vi "SeCrTs-Obtain Message Queue_R.vi"(8 "error in (no error)":errorcluster) -> (0 "error out":errorcluster, 1 "Err Queue":refnum<queue>)   [LabVIEW 2022 SP3]
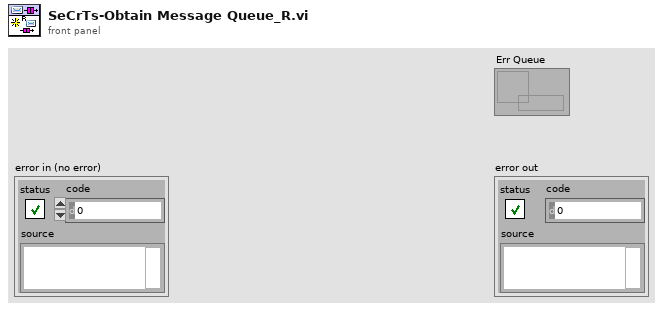
[diagram p1: front panel]
types:
  T1 = cluster{"Error Code":string, "Error Source":string}
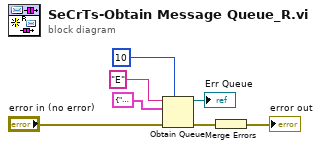
[diagram p0: block diagram]
diagram:
  n1 = Obtain Queue(max queue size (-1, unlimited)=10, name (unnamed)="E", element data type=T1 {"Error Code"="", "Error Source"=""} ("element"), error in (no error)="error in (no error)") -> (queue out=→"Err Queue":refnum<queue>, error out=w3:errorcluster)  [unwired: 1 in, 1 out]
  n2 = Merge Errors(w3) -> (→"error out":errorcluster)
